vi "Configure Sys (To) Mode (Normal).vi"(8 "error in (no error)":errorcluster, 9 "Period (100 msec)":dbl=0.1 format="%.6p", 11 "VISA resource name":refnum<visa-resource-name>) -> (0 "error out":errorcluster, 3 "VISA resource name out":refnum<visa-resource-name>)   [LabVIEW 2012, in "Quantum Composers 9000 Series.lvlib"]
doc: "This VI is used to configure the normal mode of operation of the system timer (To)."
uses:
  Quantum Composers 9000 Series.lvlib
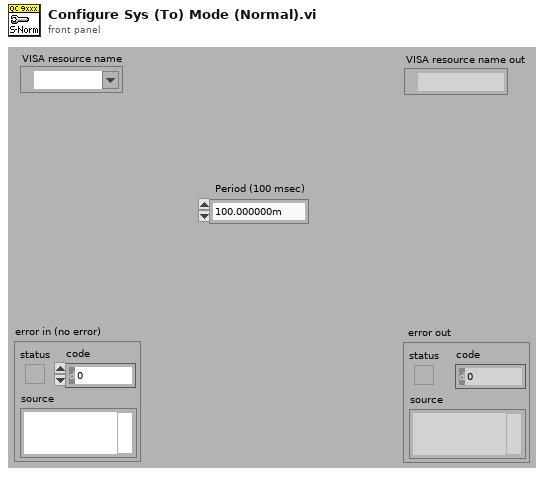
[diagram p1: front panel]
types:
  T1 = enum16{"Normal", "Single", "Burst", "Duty Cycle"}
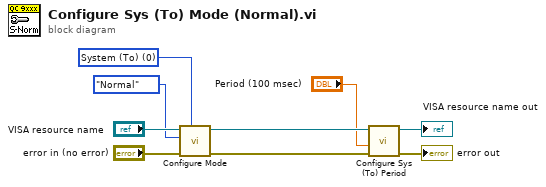
[diagram p0: block diagram]
diagram:
  w2 = 0 items=["System (To)", "Channel A", "Channel B", "Channel C", "Channel D", "Channel E", "Channel F", "Channel G", "Channel H"] ("Channel (1:Chan A)")
  n1 = call "Configure Mode.vi"("Channel (1:Chan A)"=w2, "error in (no error)"="error in (no error)", "Mode (0:Normal)"=T1."Normal" ("Chan Mode"), "VISA resource name"="VISA resource name") -> ("error out"=w6:errorcluster, "VISA resource name out"=w7:refnum<visa-resource-name>)  [unwired: 6 in]
  n2 = call "Configure Sys (To) Period.vi"("error in (no error)"=w6, "Period (100 msec)"="Period (100 msec)", "VISA resource name"=w7) -> ("error out"=→"error out":errorcluster, "VISA resource name out"=→"VISA resource name out":refnum<visa-resource-name>)  [unwired: 7 in]
